vi "CRYWait Close Step.vi"(10 "vi reference":refnum<vi>) -> ()   [LabVIEW 2013]
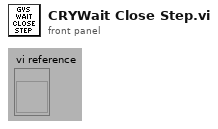
[diagram p1: front panel]
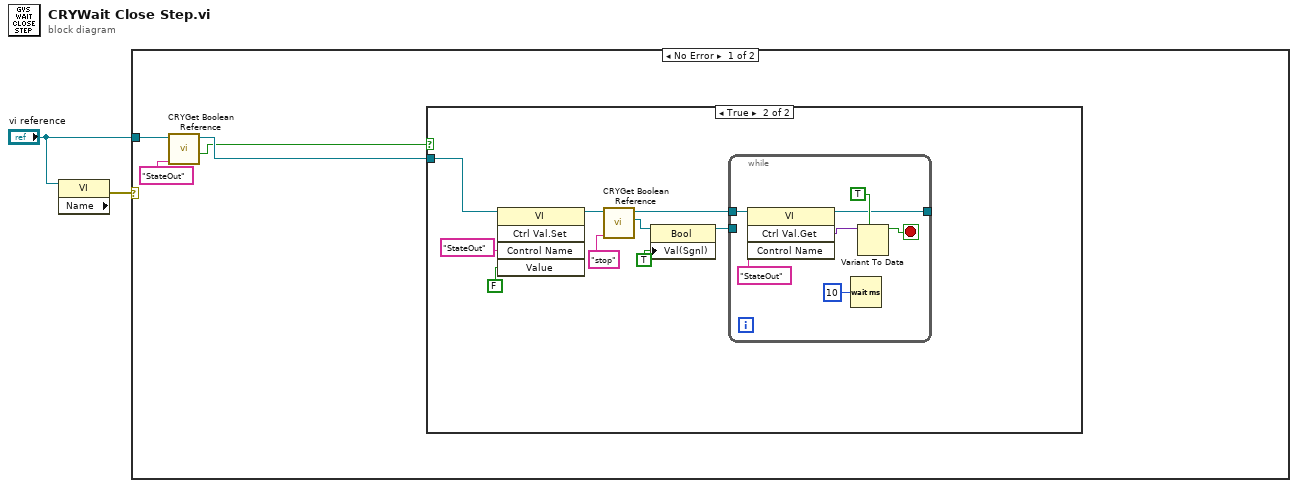
[diagram p0: block diagram]
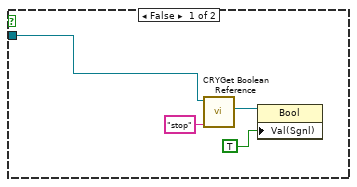
[diagram p2: hidden frame]
diagram:
  n1 = property class="VI" props=["Name"](reference="vi reference") -> (error out=w2:errorcluster)  [unwired: 1 in, 2 out]
  n2 = case shown="No Error" w2 {
    tunnel: "vi reference" -> [w3 _]
    frame No Error {
      n3 = call "CRYGet Boolean Reference.vi"("Label Name"="StateOut", "VI Refnum"=w3) -> ("Exist?"=w4:bool, "VI Refnum Out"=w5:refnum<vi>)  [unwired: 7 in, 1 out]
      n4 = case shown="True" w4 {
        tunnel: w5 -> [w10 w12]
        frame False {
          n5 = call "CRYGet Boolean Reference.vi"("Label Name"="stop", "VI Refnum"=w10) -> ("Boolean Ref"=w9:refnum<vi>)  [unwired: 7 in, 2 out]
          n6 = property class="Bool"(reference=w9, "Val(Sgnl)"=TRUE) -> ()  [unwired: 1 in, 2 out]
        }
        frame True {
          n7 = invoke class="VI" method="Ctrl Val.Set"(reference=w12, "Control Name"="StateOut", "Value"=FALSE) -> (reference out=w14:refnum<vi>)  [unwired: 2 in, 4 out]
          n8 = call "CRYGet Boolean Reference.vi"("Label Name"="stop", "VI Refnum"=w14) -> ("Boolean Ref"=w17:refnum<vi>, "VI Refnum Out"=w13:refnum<vi>)  [unwired: 7 in, 1 out]
          n9 = property class="Bool"(reference=w17, "Val(Sgnl)"=TRUE) -> (reference out=w11:refnum<vi>)  [unwired: 1 in, 1 out]
          n10 = while {
            tunnel: w13 -> [w25]
            tunnel: [w21] -> _
            tunnel: w11 -> [_]
            stop <- w22 stop-if-true
            n11 = invoke class="VI" method="Ctrl Val.Get"(reference=w25, "Control Name"="StateOut") -> (reference out=w21:refnum<vi>, "Get Control Value Variant"=w24:variant)  [unwired: 2 in, 2 out]
            n12 = Wait (ms)(milliseconds to wait=u32 10) -> ()  [unwired: 1 out]
            n13 = Variant To Data(type=TRUE, Variant=w24) -> (data=w22:bool)  [unwired: 1 in, 1 out]
          }
        }
      }
    }
    frame Error {
    }
  }
